vi "users format record from POST.vi"(8 "error in (no error)":errorcluster, 9 "Edited User (none)":T1, 10 "Current User (none)":T1, 11 "POST (empty)":T2) -> (0 "error out":errorcluster, 1 "Record to Commit":T1, 2 "Current User Credential Change?":bool, 3 "Current Record Edit?":bool)   [LabVIEW 2011]
uses:
  Addons/internet/utils/keyedarr.llb/Keyed Array.ctl
  server/database/Users/User Record.ctl
  Addons/internet/utils/strutil.llb/Case Matching.ctl
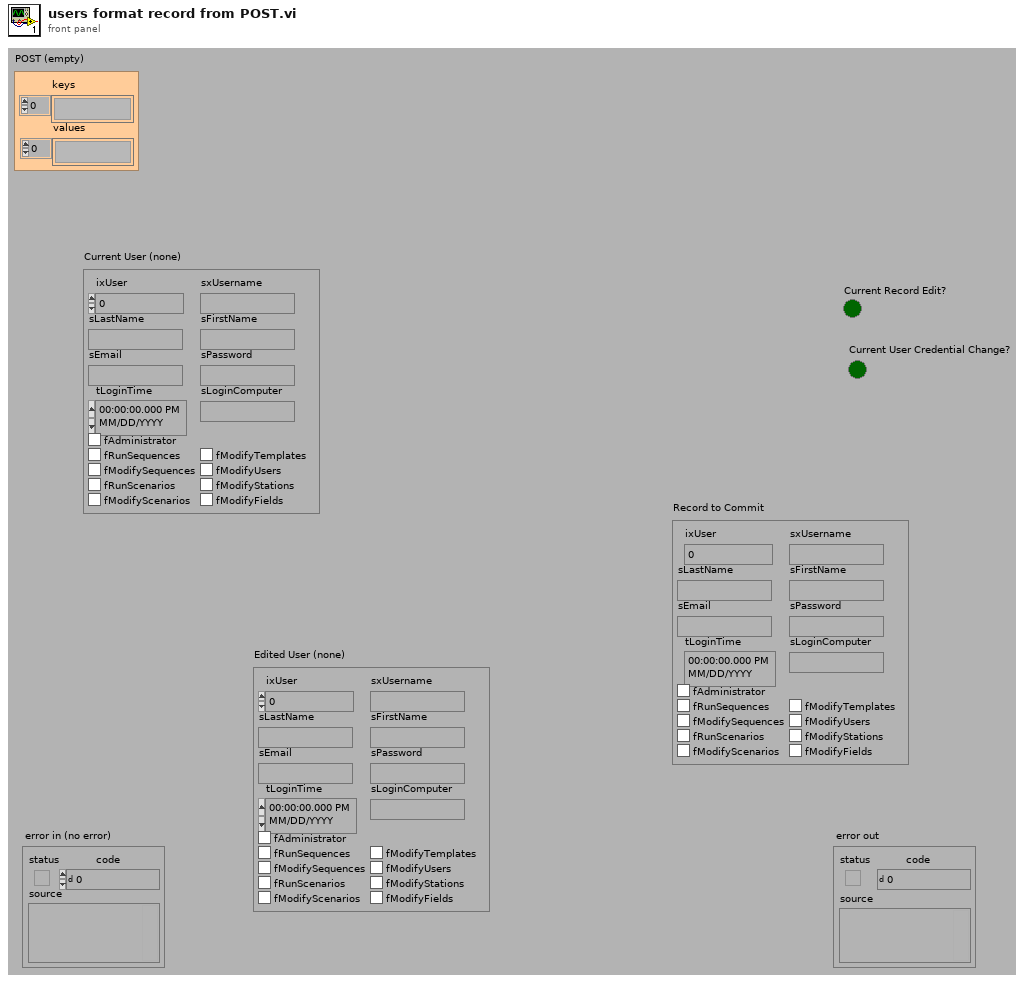
[diagram p1: front panel]
types:
  T1 = typedef "User Record.ctl" = cluster{"ixUser":i32, "sxUsername":string, "sLastName":string, "sFirstName":string, "sEmail":string, "sPassword":string, "tLoginTime":timestamp, "sLoginComputer":string, "fAdministrator":bool, "fRunSequences":bool, "fModifySequences":bool, "fRunScenarios":bool, "fModifyScenarios":bool, "fModifyTemplates":bool, "fModifyUsers":bool, "fModifyStations":bool, "fModifyFields":bool}
  T2 = typedef "Keyed Array.ctl" = cluster{"keys":string[], "values":string[]}
  T3 = typedef "Case Matching.ctl" = enum16{"a != A", "a == A", "system"}
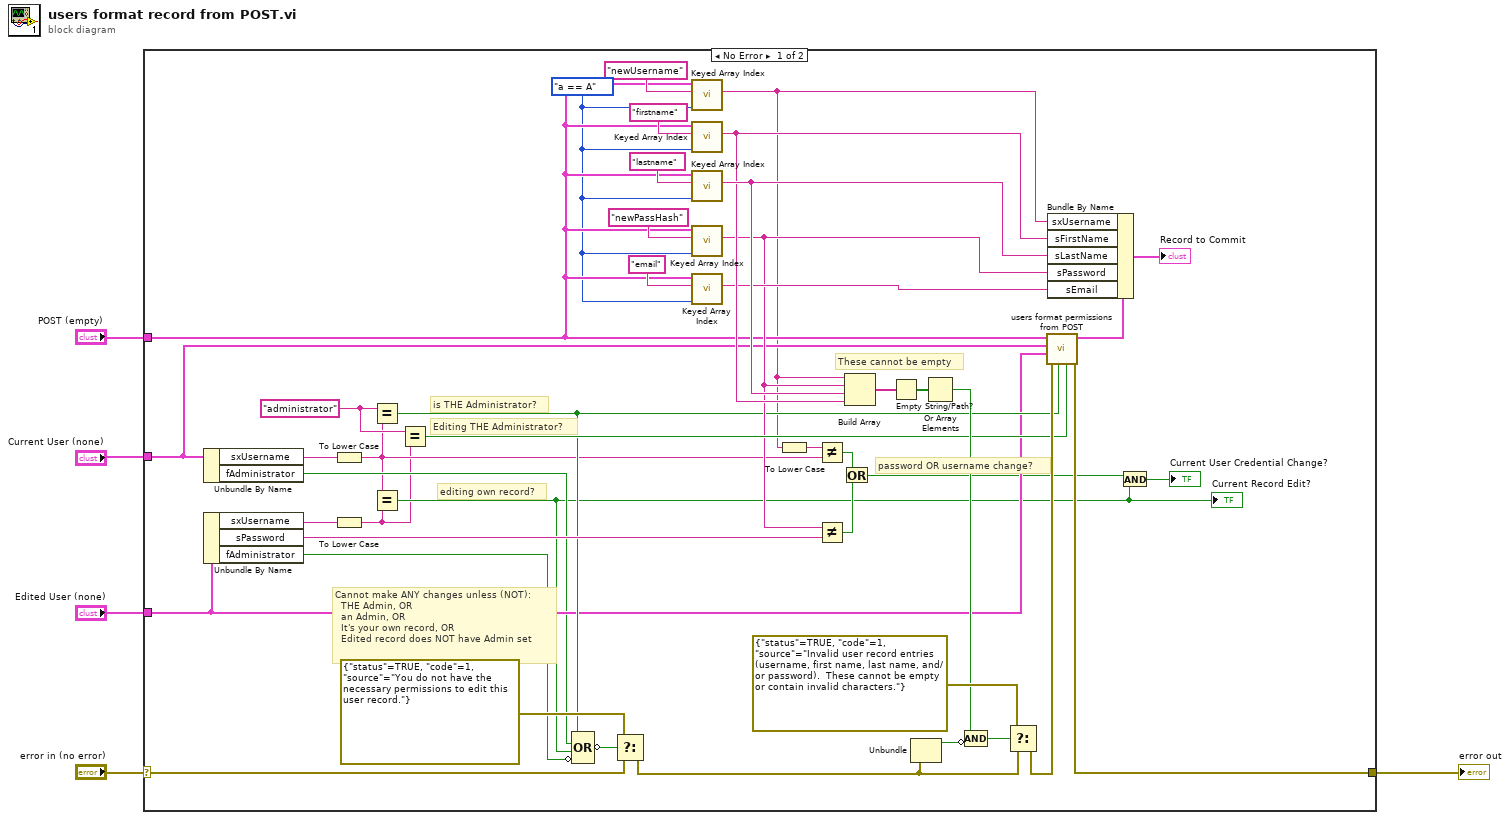
[diagram p0: block diagram]
diagram:
  n1 = case shown="No Error" "error in (no error)" {
    selector: "error in (no error)" -> [w30 w50]
    tunnel: "Current User (none)" -> [w21 _]
    tunnel: "POST (empty)" -> [w15 _]
    tunnel: "Edited User (none)" -> [w20 _]
    tunnel: [w26 w50] -> w1
    frame No Error {
      w14 = Case_Matching."a == A" ("case matching (sensitive)")
      w25 = "administrator"
      # "Editing THE Administrator?"
      # "Cannot make ANY changes unless (NOT):\n  THE Admin, OR\n  an Admin, OR\n  It's your own record, OR\n  Edited record does NOT have Admin set"
      # "These cannot be empty"
      # "password OR username change?"
      # "editing own record?"
      # "is THE Administrator?"
      n2 = Unbundle By Name(w21) -> ("sxUsername"=w45:string, "fAdministrator"=w17:bool)
      n3 = Unbundle By Name(w20) -> ("sxUsername"=w43:string, "sPassword"=w44:string, "fAdministrator"=w18:bool)
      n4 = To Lower Case(string=w45) -> (all lower case string=w13:string)
      n5 = To Lower Case(string=w43) -> (all lower case string=w7:string)
      n6 = Equal?(x=w25, y=w13) -> (x = y?=w22:bool)
      n7 = Equal?(x=w13, y=w7) -> (x = y?=w10:bool)
      "Current Record Edit?" <- w10
      n8 = Equal?(x=w25, y=w7) -> (x = y?=w24:bool)
      n9 = Compound Arithmetic op=OR(w22, w17, w10, invert w18) -> (invert w31:bool)
      n10 = Select(t=errorcluster {"status"=TRUE, "code"=1, "source"="You do not have the necessary permissions to edit this user record."}, s=w31, f=w30) -> (s? t:f=w29:errorcluster)
      n11 = call "Keyed Array Index.vi"("case matching (sensitive)"=w14, "key"="newUsername", "array in"=w15) -> ("value"=w8:string)  [unwired: 1 in, 3 out]
      n12 = call "Keyed Array Index.vi"("case matching (sensitive)"=w14, "key"="firstname", "array in"=w15) -> ("value"=w39:string)  [unwired: 1 in, 3 out]
      n13 = call "Keyed Array Index.vi"("case matching (sensitive)"=w14, "key"="lastname", "array in"=w15) -> ("value"=w40:string)  [unwired: 1 in, 3 out]
      n14 = call "Keyed Array Index.vi"("case matching (sensitive)"=w14, "key"="newPassHash", "array in"=w15) -> ("value"=w23:string)  [unwired: 1 in, 3 out]
      n15 = call "Keyed Array Index.vi"("case matching (sensitive)"=w14, "key"="email", "array in"=w15) -> ("value"=w36:string)  [unwired: 1 in, 3 out]
      n16 = To Lower Case(string=w8) -> (all lower case string=w6:string)
      n17 = Not Equal?(x=w6, y=w13) -> (x != y?=w12:bool)
      n18 = Not Equal?(x=w23, y=w44) -> (x != y?=w11:bool)
      n19 = Or(x=w12, y=w11) -> (x .or. y?=w9:bool)
      n20 = Build Array(w8, w23, w40, w39) -> (w38:string[])
      n21 = Empty String/Path?(string/path=w38) -> (empty?=w37:bool[])
      n22 = Unbundle(w29) -> ("status"=w34:bool)  [unwired: 2 out]
      n23 = Or Array Elements(Boolean array=w37) -> (logical OR=w32:bool)
      n24 = Compound Arithmetic op=AND(w32, invert w34) -> (w33:bool)
      n25 = Select(t=errorcluster {"status"=TRUE, "code"=1, "source"="Invalid user record entries (username, first name, last name, and/or password).  These cannot be empty or contain invalid characters."}, s=w33, f=w29) -> (s? t:f=w27:errorcluster)
      n26 = call "users format permissions from POST.vi"("Edit Admin? (f)"=w24, "THE Admin? (f)"=w22, "error in (no error)"=w27, "Permissions to Edit (F)"=w20, "Current User Permissions (F)"=w21, "POST (empty)"=w15) -> ("error out"=w26:errorcluster, "User Record"=w19:T1)  [unwired: 4 out]
      n27 = Bundle By Name(cluster=w19, "sxUsername"=w8, "sFirstName"=w39, "sLastName"=w40, "sPassword"=w23, "sEmail"=w36) -> (→"Record to Commit":T1)
      n28 = And(x=w9, y=w10) -> (x .and. y?=→"Current User Credential Change?":bool)
    }
    frame Error {
    }
  }
  "error out" <- w1
